vi "T calibration.vi"() -> ()   [LabVIEW 2019]
uses:
  <vilib>/Analysis/polynomials.llb/1D Polynomial Evaluation (DBL).vi
  <vilib>/Analysis/NI_AALPro.lvlib
panel:
  out "Waveform Graph":dbl[](graph)
  in  "End R":dbl=60.0
  in  "Start R":dbl=40.0
  out "XY Graph":cluster{dbl[], "P(A)":dbl[]}(graph)
  in  "Log T to Log R":dbl[](array[numeric])=[26587.18102, -78446.79509, 92571.02475, -54604.91141, 16100.55137, -1898.43152] format="%#_13g"
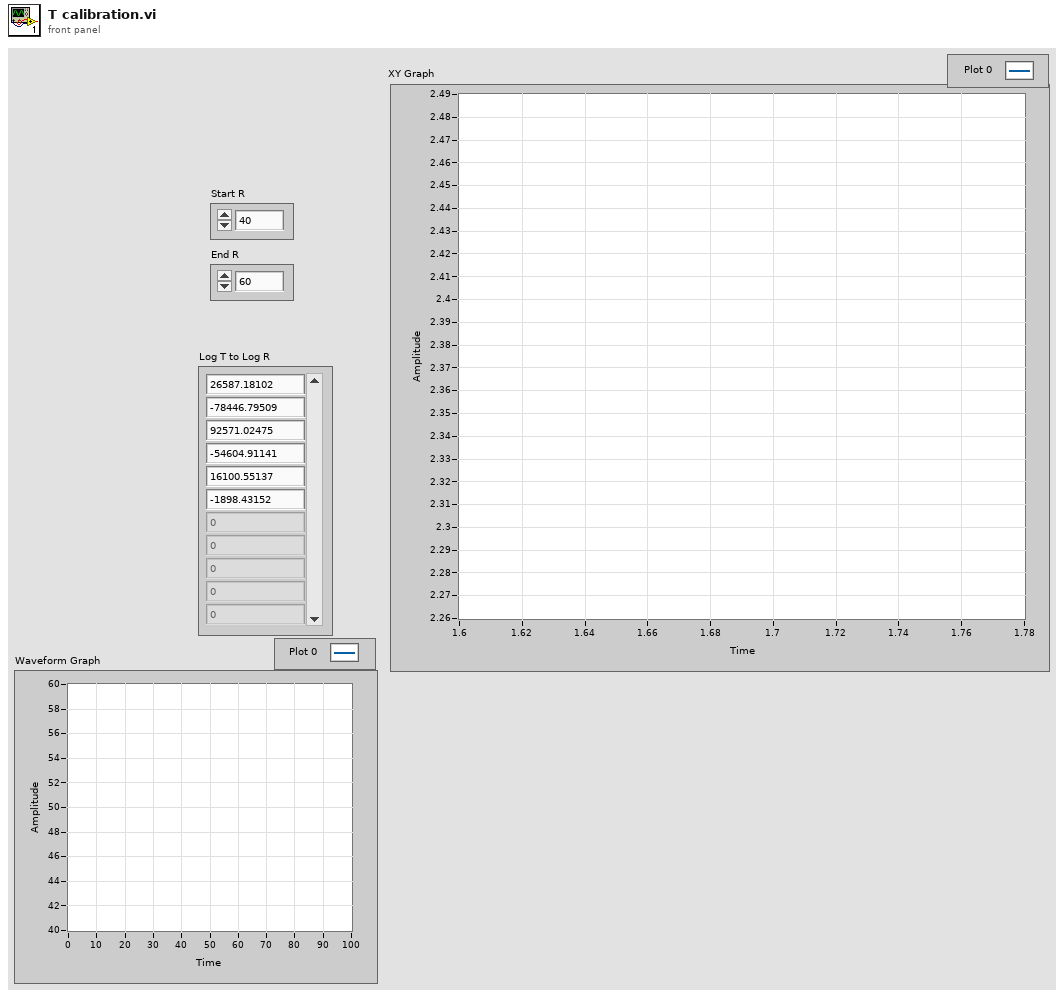
[diagram p1: front panel]
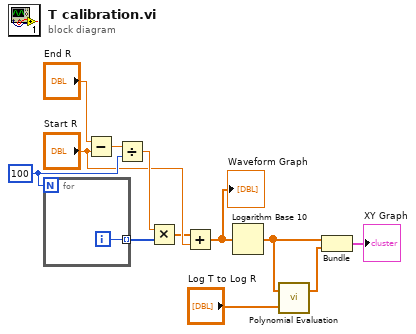
[diagram p0: block diagram]
diagram:
  w10 = 100
  n1 = for {
    N: w10 -> [_]
    tunnel: [w13] -> w8 mode=indexing
    i -> [w13]
  }
  n2 = Subtract(x="End R", y="Start R") -> (x-y=w11:dbl)
  n3 = Divide(x=w11, y=w10) -> (x/y=w9:dbl)
  n4 = Multiply(x=w9, y=w8) -> (x*y=w6:dbl[])
  n5 = Add(x=w6, y="Start R") -> (x+y=w5:dbl[])
  "Waveform Graph" <- w5
  n6 = Logarithm Base 10(1:w5) -> (0:w3:dbl[])
  n7 = call-poly <vilib>:"Polynomial Evaluation.vi"("P(x)"="Log T to Log R", "A"=w3) -> ("P(A)"=w2:dbl[])  [unwired: 1 out]
  n8 = Bundle(w3, "P(A)"=w2) -> (→"XY Graph":cluster{dbl[], "P(A)":dbl[]})  [unwired: 1 in]
